vi "Read Config.vi"(8 "error in (no error)":errorcluster, 9 "Re-Init?":bool, 10 "ICM File In":path, 11 "Multiple Queries in":refnum<class "Multiple Queries.lvclass">) -> (0 "error out":errorcluster, 3 "Multiple Queries out":refnum<class "Multiple Queries.lvclass">)   [LabVIEW 2024, in "Multiple Queries.lvclass"]
doc: "Multiple Queries.lvclass:Read Config.vi\n\nThis VI reads the configuration data for the Multple Queries child class.\n\nInstrument Communication Module Version 1.0\nDecember, 2017 Original Code Consulting David Thomson\n www.originalcode.com"
uses:
  Multiple Queries.lvclass
  Multiple Queries.lvclass/Multiple Queries.ctl
  Query/Query.lvclass
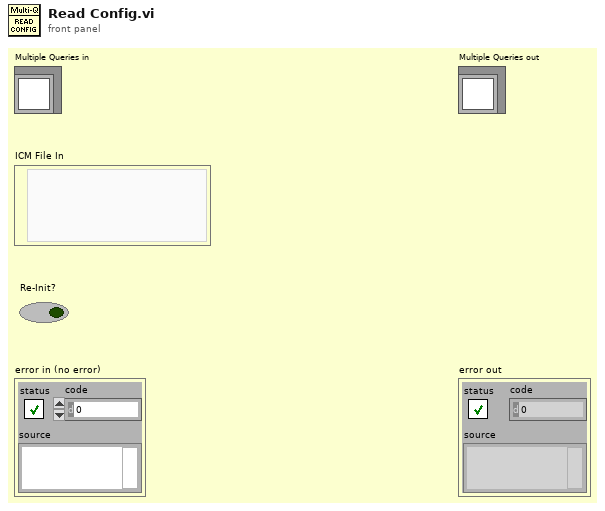
[diagram p1: front panel]
types:
  T1 = typedef "Multiple Queries.lvclass/Multiple Queries Config.ctl" = cluster{"Queries":string[], "Time Between Queries (ms)":u32, "Response Separator":string}
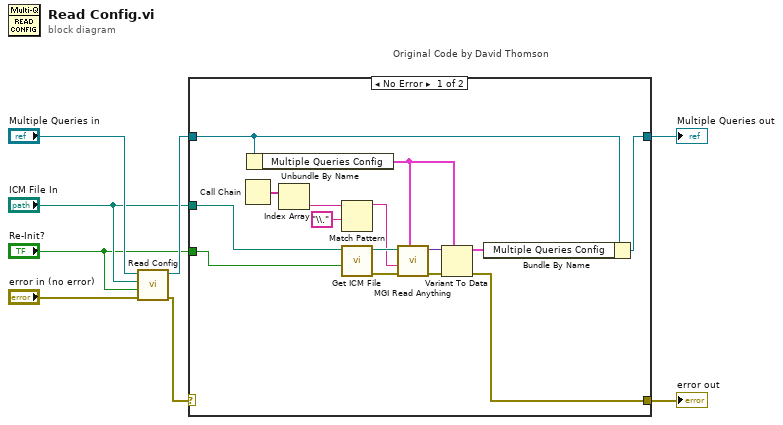
[diagram p0: block diagram]
diagram:
  n1 = call-parent "Read Config.vi"("error in (no error)"="error in (no error)", "Re-Init?"="Re-Init?", "ICM File In"="ICM File In", "Query in"="Multiple Queries in") -> ("error out"=w6:errorcluster, "Query out"=w3:refnum<class "Multiple Queries.lvclass">)  [unwired: 6 in]
  n2 = case "Original Code by David Thomson" shown="No Error" w6 {
    selector: w6 -> [_ w25]
    tunnel: [w15 w25] -> w5
    tunnel: [w12 w24] -> w4
    tunnel: w3 -> [w11 w24]
    tunnel: "ICM File In" -> [w10 _]
    tunnel: "Re-Init?" -> [w9 _]
    frame No Error {
      n3 = Call Chain() -> (call chain=w20:string[])
      n4 = Unbundle By Name(w11) -> ("Multiple Queries Config"=w13:T1)
      n5 = Index Array(array=w20) -> (element=w21:string)  [unwired: 1 in]
      n6 = Match Pattern(string=w21, regular expression="\\.") -> (before substring=w18:string)  [unwired: 1 in, 3 out]
      n7 = call "Get ICM File.vi"("Re-Init?"=w9, "ICM File In"=w10) -> ("error out"=w22:errorcluster, "ICM File"=w23:path)  [unwired: 8 in]
      n8 = call "MGI Read Anything.vi"("Type of Anything"=w13, "Error In"=w22, "Section Name (Name of \"Type of Anything\")"=w18, "Path (dialog)"=w23) -> ("Error Out"=w16:errorcluster, "Anything"=w17:variant)  [unwired: 4 in, 2 out]
      n9 = Variant To Data(error in=w16, type=w13, Variant=w17) -> (data=w14:T1, error out=w15:errorcluster)
      n10 = Bundle By Name(cluster=w11, "Multiple Queries Config"=w14) -> (w12:refnum<class "Multiple Queries.lvclass">)
    }
    frame Error {
    }
  }
  "error out" <- w5
  "Multiple Queries out" <- w4
